vi "_Remote Reboot.vi"(0 "IP Address":string) -> (1 "Connected":bool)   [LabVIEW 2015]
uses:
  Type/_RT Instrument State.ctl
  Type/_RT Command.ctl
  Configuration/_Global Configuration.vi
  <vilib>/nisyscfg/nisyscfg.lvlib
panel:
  in  "stop":bool
  out "Current MS Status":T1
  in  "error in (no error)":errorcluster
  # "Please wait a few minutes while rebooting the embedded PC"
  # "(This dialog will automatically close when rebooting is finished)"
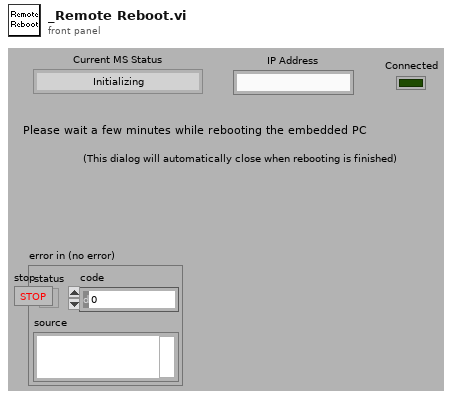
[diagram p1: front panel]
types:
  T1 = typedef "_RT Instrument State.ctl" = enum16{"Initializing", "Mass Spectrometer is Off", "Starting Up", "Turning Power Off", "Going to Standby", "Roughing Pump Ready", "Turning Turbo Off", "Turbo Startup", "Turbopump Ready", "Checking Vacuum", "Going to Ready", "Ready", "Running", "Source Standby", "Lost Communication", "Shutting Down", "Fault", "24V Standby", "Go to 24V Standby", "Turbopump Ready-Waiting"}
  T2 = typedef "_RT Command.ctl" = enum16{"Start", "StartActualRun", "Stop", "Runtime Update", "Get Data", "Get Info", "Get Status", "Get Param", "Get Config", "Get Table", "Read ADC", "Set Oscillator", "Update Config", "Update Table", "Set All Pol", "Set Pol and DC", "Set Max Mass", "Toggle RP", "Toggle EL", "Set PIC", "Initialize Turbo", "Send Turbo Comm", "Close Turbo", "P1", "P2", "P3", "Send Serial", "Set LC Out", "Get LC In", "Read VAC", "Test Table", "Toggle Power", "Get Startup", "Set Startup", "Get ADC Table", "Set ADC Table", "Get Brief Status", "Get Detail Status", "Auxiliary Update", "Set CC Logics", "Set CC Input Logics", "Ignore Error"}
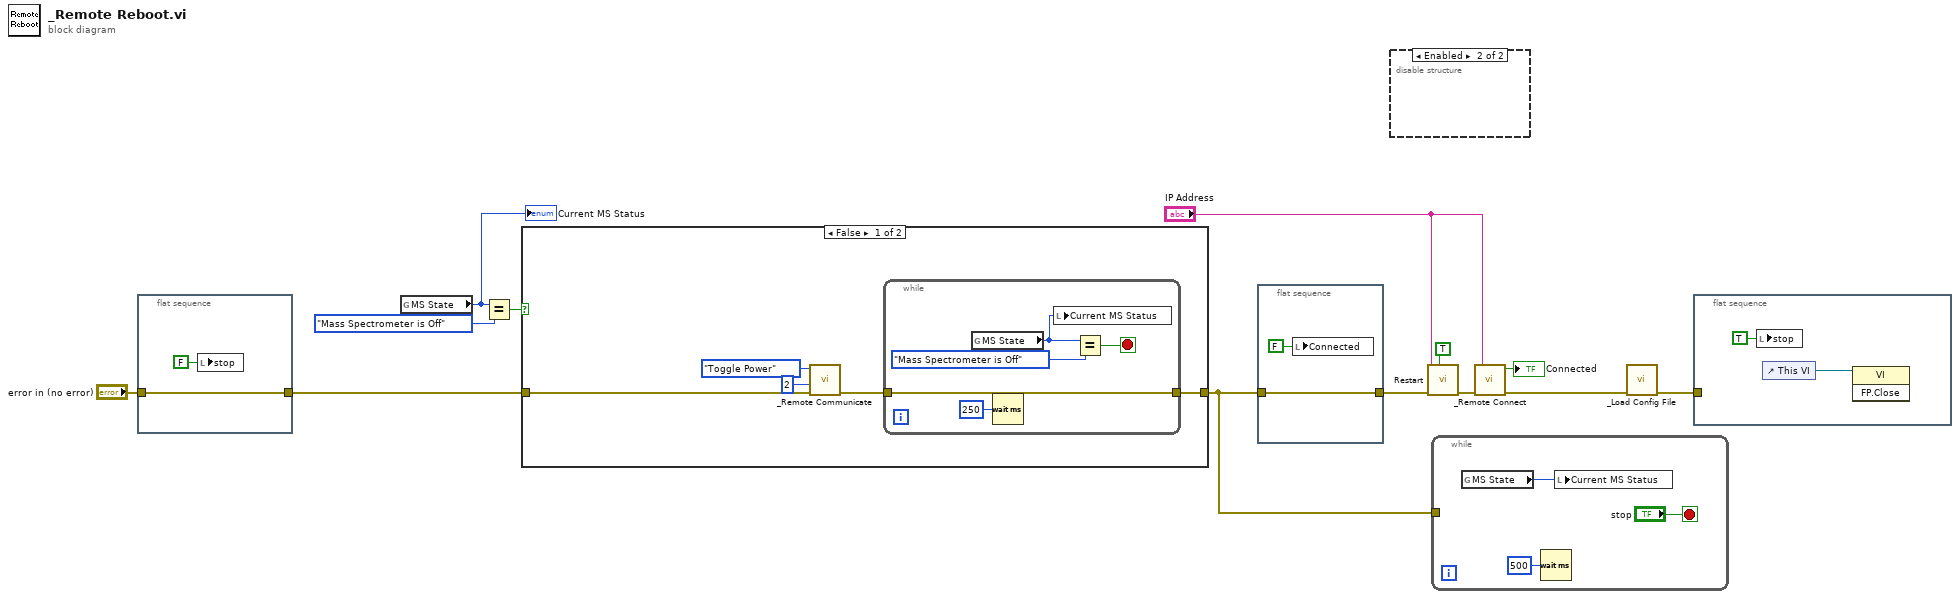
[diagram p0: block diagram]
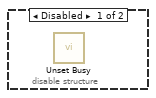
[diagram p2: hidden frame]
diagram:
  n1 = flat-sequence {
    tunnel: "error in (no error)" -> [w14]
    tunnel: [w14] -> w3
    frame #0 {
      n2 = local write "stop"(FALSE ("stop")) -> ()
    }
  }
  n3 = global read "_Global Configuration.vi" "MS State"() -> (w6:T1)
  "Current MS Status" <- w6
  n4 = Equal?(x=w6, y=_RT_Instrument_State."Mass Spectrometer is Off") -> (x = y?=w7:bool)
  n5 = case shown="False" w7 {
    tunnel: [w16 w26] -> w1
    tunnel: w3 -> [w18 w26]
    frame False {
      n6 = call "_Remote Communicate.vi"("error in (no error)"=w18, "DC Param"=u16 2, "Command"=_RT_Command."Toggle Power") -> ("error out"=w17:errorcluster)  [unwired: 3 in, 3 out]
      n7 = while {
        tunnel: w17 -> [w23]
        tunnel: [w23] -> w16
        stop <- w24 stop-if-true
        n8 = global read "_Global Configuration.vi" "MS State"() -> (w21:T1)
        n9 = Wait (ms)(milliseconds to wait=u32 250) -> ()  [unwired: 1 out]
        n10 = local write "Current MS Status"(w21) -> ()
        n11 = Equal?(x=w21, y=_RT_Instrument_State."Mass Spectrometer is Off") -> (x = y?=w24:bool)
      }
    }
    frame True {
    }
  }
  n12 = flat-sequence {
    tunnel: [w28] -> w2
    tunnel: w1 -> [w28]
    frame #0 {
      n13 = local write "Connected"(FALSE ("Connected")) -> ()
    }
  }
  n14 = disable-structure shown="Enabled" {
    frame Disabled {
      n15 = call <vilib>:"Unset Busy.vi"() -> ()  [unwired: 2 in, 10 out]
    }
    frame Enabled {
    }
  }
  n16 = call <vilib>:"Restart.vi"("Wait Until Complete (T)"=TRUE, "error in (no error)"=w2, "Session in"="IP Address") -> ("error out"=w9:errorcluster)  [unwired: 6 in, 2 out]
  n17 = while {
    tunnel: w1 -> [_]
    stop <- "stop" stop-if-true
    n18 = global read "_Global Configuration.vi" "MS State"() -> (w30:T1)
    n19 = Wait (ms)(milliseconds to wait=u32 500) -> ()  [unwired: 1 out]
    n20 = local write "Current MS Status"(w30) -> ()
  }
  n21 = call "_Remote Connect.vi"("error in (no error)"=w9, "IP Address"="IP Address") -> ("error out"=w13:errorcluster, "TCP"=→"Connected":bool)  [unwired: 4 out]
  n22 = call "_Load Config File.vi"("error in (no error)"=w13) -> ("error out"=w5:errorcluster)  [unwired: 6 out]
  n23 = flat-sequence {
    tunnel: w5 -> [_]
    frame #0 {
      n24 = local write "stop"(TRUE ("stop")) -> ()
      n25 = control-ref of="This VI"() -> (w32:refnum<vi>)
      n26 = invoke class="VI" method="FP.Close"(reference=w32) -> ()  [unwired: 2 in, 3 out]
    }
  }
